vi "PreBuild.vi"(8 "error in (no error)":errorcluster, 11 "Build in":refnum<class "AB_Build.lvclass">) -> (0 "error out":errorcluster, 3 "Build out":refnum<class "AB_Build.lvclass">)   [LabVIEW 2020, in "AB_Build.lvclass"]
uses:
  <vilib>/AppBuilder/AB_Classes/Build/AB_Build.lvclass
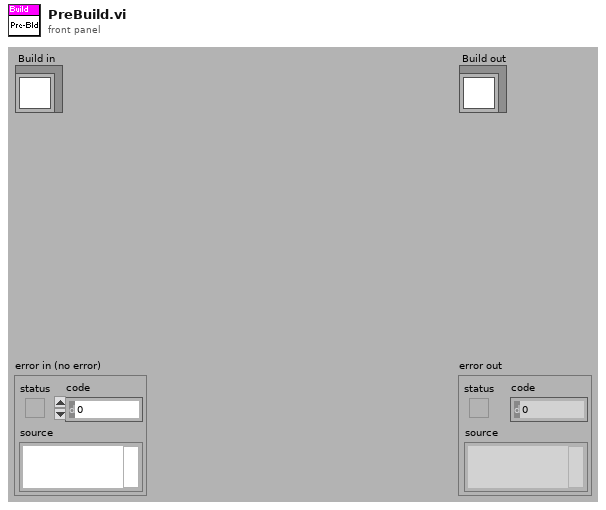
[diagram p1: front panel]
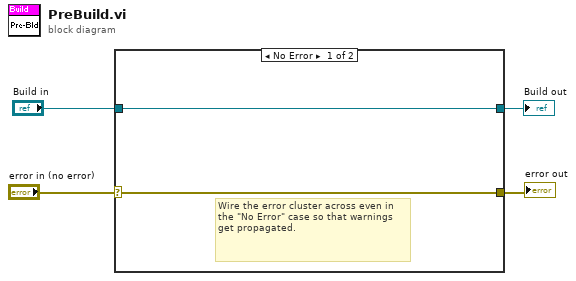
[diagram p0: block diagram]
diagram:
  n1 = case shown="No Error" "error in (no error)" {
    selector: "error in (no error)" -> [w5 w8]
    tunnel: [w5 w8] -> w3
    tunnel: [w6 w7] -> w1
    tunnel: "Build in" -> [w6 w7]
    frame No Error {
      # "Wire the error cluster across even in the \"No Error\" case so that warnings get propagated."
    }
    frame Error {
    }
  }
  "error out" <- w3
  "Build out" <- w1
